vi "Write Nested Queue.vi"(8 "error in (no error)":errorcluster, 9 "Tester Enqueuer":refnum<class "Message Enqueuer.lvclass">, 10 "Nested Name":string, 11 "Generic Actor in":refnum<class "Generic Actor.lvclass">) -> (0 "error out":errorcluster, 3 "Generic Actor out":refnum<class "Generic Actor.lvclass">)   [LabVIEW 2020, in "Generic Actor.lvlib" / "Generic Actor.lvclass"]
uses:
  Generic Actor.lvclass
  <vilib>/ActorFramework/Message Enqueuer/Message Enqueuer.lvclass
  Generic Actor.lvclass/Generic Actor.ctl
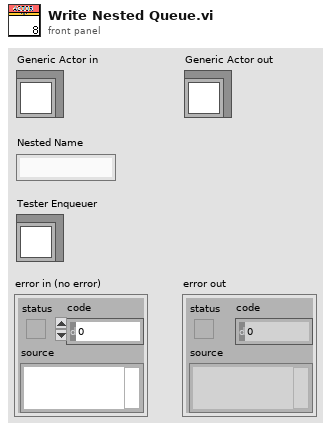
[diagram p1: front panel]
types:
  T1 = map{string, refnum<class "Message Enqueuer.lvclass">}
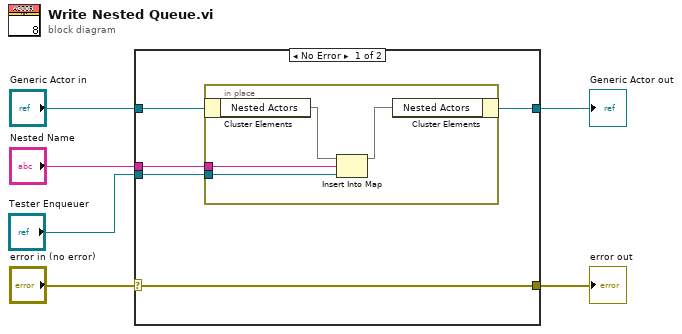
[diagram p0: block diagram]
diagram:
  n1 = case shown="No Error" "error in (no error)" {
    selector: "error in (no error)" -> [w11 w17]
    tunnel: [w11 w17] -> w5
    tunnel: [w9 w16] -> w3
    tunnel: "Generic Actor in" -> [w10 w16]
    tunnel: "Nested Name" -> [w8 _]
    tunnel: "Tester Enqueuer" -> [w7 _]
    frame No Error {
      n2 = in-place {
        in-place-border: w8 -> [w13]
        in-place-border: w7 -> [w12]
        n3 = in-place-cluster #1(w10) -> ("Nested Actors"=w15:T1)
        n4 = Insert Into Map(map in=w15, key=w13, value=w12) -> (map out=w14:T1)  [unwired: 2 out]
        n5 = in-place-cluster #1("Nested Actors"=w14) -> (w9:refnum<class "Generic Actor.lvclass">)
      }
    }
    frame Error {
    }
  }
  "error out" <- w5
  "Generic Actor out" <- w3
